vi "parse_retrieve_point_response.vi"(8 "error in (no error)":errorcluster, 10 "body":string, 11 "headers":string) -> (0 "error out":errorcluster, 3 "vector":T1)   [LabVIEW 2020, in "vector_qdrant.lvclass"]
uses:
  vector_qdrant.lvclass
  abstract_vector_base/vector.ctl
  abstract_vector_base/abstract_vector_base.lvclass
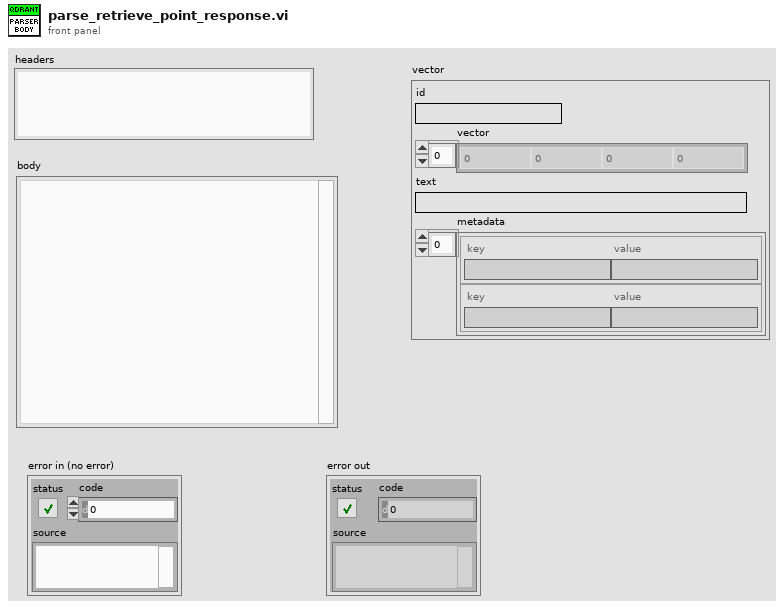
[diagram p1: front panel]
types:
  T1 = typedef "abstract_vector_base.lvclass/vector.ctl" = cluster{"id":string, "vector":dbl[], "text":string, "metadata":cluster{"key":string, "value":string}[]}
  T2 = cluster{"id":string, "payload":cluster{"text":string}, "vector":dbl[]}
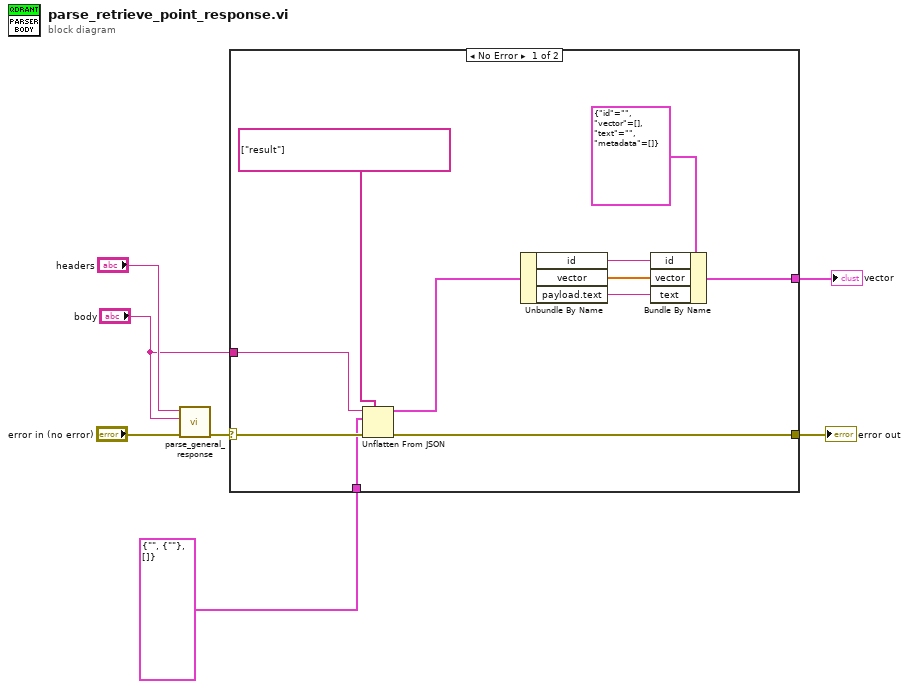
[diagram p0: block diagram]
diagram:
  n1 = call "parse_general_response.vi"("error in (no error)"="error in (no error)", "body"="body", "headers"="headers") -> ("error out"=w5:errorcluster)  [unwired: 8 in]
  n2 = case shown="No Error" w5 {
    selector: w5 -> [w18 w19]
    tunnel: [w15 w19] -> w7
    tunnel: "body" -> [w16 _]
    tunnel: T2 {"id"="", "payload"={"text"=""}, "vector"=[]} -> [w14 _]
    tunnel: [w12 _] -> w1
    frame No Error {
      n3 = Unflatten From JSON(path=string[] ["result"], JSON string=w16, type and defaults=w14, error in (no error)=w18) -> (value=w13:T2, error out=w15:errorcluster)  [unwired: 3 in]
      n4 = Unbundle By Name(w13) -> ("id"=w11:string, "vector"=w10:dbl[], "payload.text"=w9:string)
      n5 = Bundle By Name(cluster=T1 {"id"="", "vector"=[], "text"="", "metadata"=[]} ("vector"), "id"=w11, "vector"=w10, "text"=w9) -> (w12:T1)
    }
    frame Error {
    }
  }
  "error out" <- w7
  "vector" <- w1
